vi "bump disorder.vi"(5 "length percent":dbl=1.0, 7 "begin percent":dbl=1.0, 8 "error in":errorcluster, 9 "amp":dbl=1.0, 10 "level":dbl=1.0, 11 "Points":i32=10) -> (0 "error out":errorcluster, 3 "disorder":dbl[](array[numeric]))   [LabVIEW 2023]
uses:
  <vilib>/gmath/NI_Gmath.lvlib
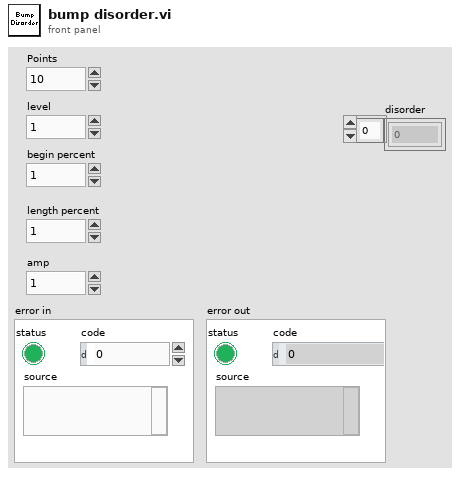
[diagram p1: front panel]
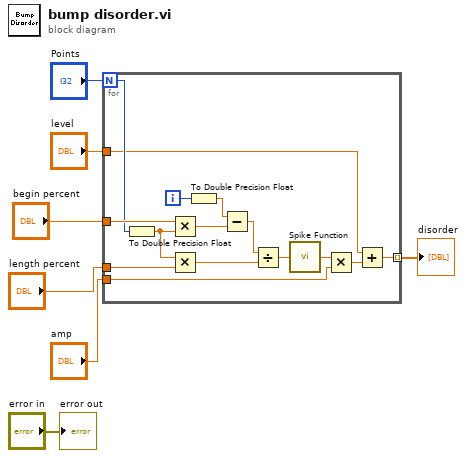
[diagram p0: block diagram]
diagram:
  n1 = for {
    N: "Points" -> [w20]
    tunnel: [w8] -> w6 mode=indexing
    tunnel: "begin percent" -> [w22]
    tunnel: "length percent" -> [w15]
    tunnel: "amp" -> [w11]
    tunnel: "level" -> [w9]
    i -> [w21]
    n2 = To Double Precision Float(number=w20) -> (double precision float=w16:dbl)
    n3 = Multiply(x=w22, y=w16) -> (x*y=w18:dbl)
    n4 = Multiply(x=w16, y=w15) -> (x*y=w14:dbl)
    n5 = To Double Precision Float(number=w21) -> (double precision float=w19:dbl)
    n6 = Subtract(x=w19, y=w18) -> (x-y=w17:dbl)
    n7 = Divide(x=w17, y=w14) -> (x/y=w13:dbl)
    n8 = call <vilib>:"Spike Function.vi"("x"=w13) -> ("spike(x)"=w12:dbl)
    n9 = Multiply(x=w12, y=w11) -> (x*y=w10:dbl)
    n10 = Add(x=w9, y=w10) -> (x+y=w8:dbl)
  }
  "disorder" <- w6
  "error out" <- "error in"
